vi "RIGOL DS1000 Series Acquire Continuous Waveform.vi"() -> ()   [LabVIEW 2018]
doc: "This example shows how to use autosetup and acquire a waveform on a single channel."
uses:
  <instrlib>/RIGOL DS1000 Series/Public/Data/Read (Single Waveform).vi
  <vilib>/Waveform/WDTFileIO.llb/Export Waveform To Spreadsheet File.vi
  <instrlib>/RIGOL DS1000 Series/RIGOL DS1000 Series.lvlib
panel:
  out "Peak to Peak":dbl
  out "Mean (DC)":dbl
  out "Numeric":i32
  out "Duty Cycle":dbl
  out "Frequency":dbl
  in  "Channel (0: Channel 1)":u16(ring) items=["Channel 1", "Channel 2", "Channel 3", "Channel 4"]
  in  "Stop":bool
  in  "Timeout (10000 ms)":u32=10000
  out "Waveform Data":waveform(dbl)(graph)
  in  "VISA resource name":refnum<visa-resource-name>
  # "(c) 2010-2012, RIGOL Technologies, Inc.  All Rights Reserved."
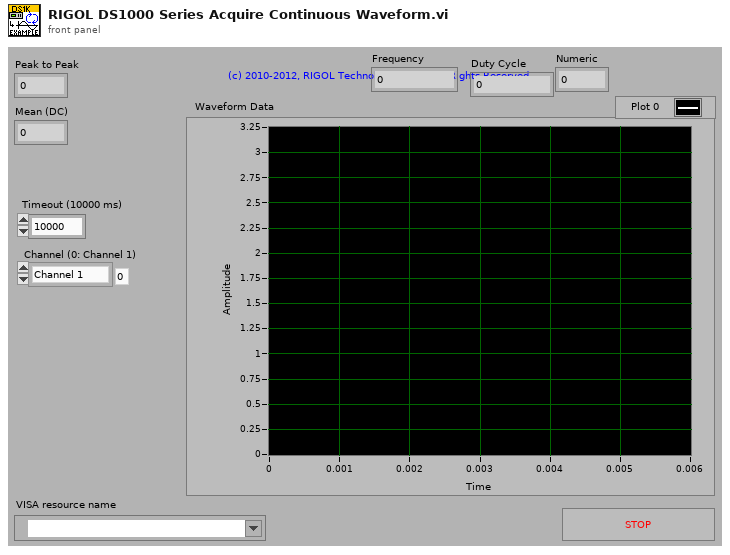
[diagram p1: front panel]
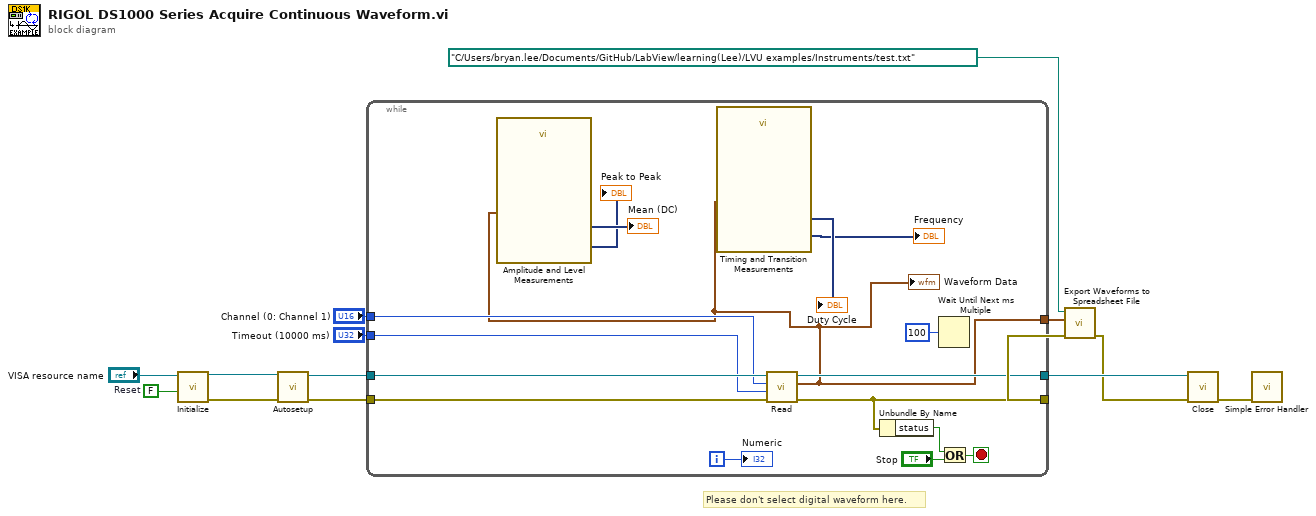
[diagram p0: block diagram]
diagram:
  w5 = FALSE  # Reset
  # "Please don't select digital waveform here."
  n1 = call <instrlib>:"Initialize.vi"("Reset (True)"=w5, "VISA resource name"="VISA resource name") -> ("error out"=w10:errorcluster, "VISA resource name out"=w9:refnum<visa-resource-name>)  [unwired: 2 in, 6 out]
  n2 = call "Autosetup.vi"("error in (no error)"=w10, "VISA resource name"=w9) -> ("error out"=w7:errorcluster, "VISA resource name out"=w8:refnum<visa-resource-name>)  [unwired: 8 in]
  n3 = while {
    tunnel: w8 -> [w30]
    tunnel: w7 -> [w29]
    tunnel: [w28] -> w13
    tunnel: [w25] -> w2
    tunnel: "Timeout (10000 ms)" -> [w21]
    tunnel: "Channel (0: Channel 1)" -> [w22]
    tunnel: [w17] -> w4
    i -> [w19]
    stop <- w26 stop-if-true
    n4 = call-poly <instrlib>:"Read.vi"("error in (no error)"=w29, "Timeout (10000 ms)"=w21, "Channel (0: Channel 1)"=w22, "VISA resource name"=w30) -> ("error out"=w25:errorcluster, "Waveform Data"=w17:waveform(dbl), "VISA resource name out"=w28:refnum<visa-resource-name>)  [unwired: 5 out]
    "Waveform Data" <- w17
    n5 = call "Amplitude and Level Measurements"("Signals"=w17) -> ("Mean (DC)"=→"Mean (DC)":dynamicdata, "Peak to Peak"=→"Peak to Peak":dynamicdata)  [unwired: 12 in, 1 out]
    n6 = call "Timing and Transition Measurements"("Signals"=w17) -> ("Frequency"=→"Frequency":dynamicdata, "Duty Cycle"=→"Duty Cycle":dynamicdata)  [unwired: 8 in, 1 out]
    n7 = Unbundle By Name(w25) -> ("status"=w24:bool)
    n8 = Wait Until Next ms Multiple(millisecond multiple=u32 100) -> ()  [unwired: 1 out]
    n9 = Or(x=w24, y="Stop") -> (x .or. y?=w26:bool)
    "Numeric" <- w19
  }
  n10 = call-poly <vilib>:"Export Waveforms to Spreadsheet File.vi"("error in (no error)"=w2, "waveform"=w4, "file path (dialog if empty)"=path "C:/Users/bryan.lee/Documents/GitHub/LabView/learning(Lee)/LVU examples/Instruments/test.txt") -> ("error out"=w1:errorcluster)  [unwired: 7 in, 1 out]
  n11 = call <instrlib>:"Close.vi"("error in (no error)"=w1, "VISA resource name"=w13) -> ("error out"=w14:errorcluster)  [unwired: 9 out]
  n12 = call <vilib>:"Simple Error Handler.vi"("error in (no error)"=w14) -> ()  [unwired: 1 in, 8 out]
